vi "Is Error.vi"(11 "jettl Event Actor in":refnum<class "jettl Event Actor.lvclass">) -> (3 "jettl Event Actor out":refnum<class "jettl Event Actor.lvclass">)   [LabVIEW 2021, in "jettl.lvlib" / "jettl Event Actor.lvclass"]
uses:
  jettl Event Actor.lvclass
  Event State/Error Event State/Error Event State.lvclass
  C:/git/jettl/src/jettl/Event State/Event State/Event State.lvclass
  jettl Event Actor.lvclass/jettl Event Actor.ctl
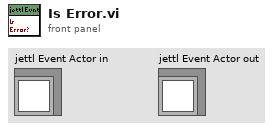
[diagram p1: front panel]
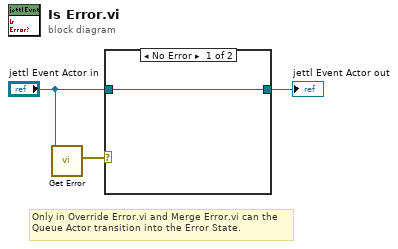
[diagram p0: block diagram]
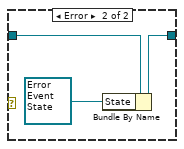
[diagram p2: hidden frame]
diagram:
  # "Only in Override Error.vi and Merge Error.vi can the Queue Actor transition into the Error State."
  n1 = call-dynamic "Get Error.vi"("jettl Event Actor in"="jettl Event Actor in") -> ("Error"=w1:errorcluster)  [unwired: 10 in]
  n2 = case shown="No Error" w1 {
    tunnel: [w4 w6] -> w3
    tunnel: "jettl Event Actor in" -> [w4 w7]
    frame No Error {
    }
    frame Error {
      n3 = Bundle By Name(cluster=w7, "State"=refnum<class "Error Event State.lvclass"> refnum ("jettl.lvlib:Error Event State.lvclass")) -> (w6:refnum<class "jettl Event Actor.lvclass">)
    }
  }
  "jettl Event Actor out" <- w3
